vi "IntPRFCount.vi"(0 "prf (kHz)":dbl=1.0 format="%.3f", 2 "prf (f)/motor (t)":bool, 9 "Divide prf by":i32=2, 13 "therapy divide by (T)":bool) -> (6 "new prf":dbl format="%.2f", 15 "Divide prf out":i32=1)   [LabVIEW 2022 SP3]
uses:
  Pulsers/PulserGlobals.vi
  Motion Controllers/-MotionRoutines/MotionGlobals.vi
  <vilib>/DAQmx/create/channels.llb/DAQmx Create Channel (CO-Pulse Generation-Ticks).vi
  <vilib>/DAQmx/create/channels.llb/DAQmx Create Channel (CO-Pulse Generation-Frequency).vi
panel:
  # "Indicates if counter 0 is is giving a 1-1 output pulse\n for each motor inpute or if it is generating a continous prf."
  # "Determines whether counter 1 is used to fire \ntherapy at some divided multiple of counter 0."
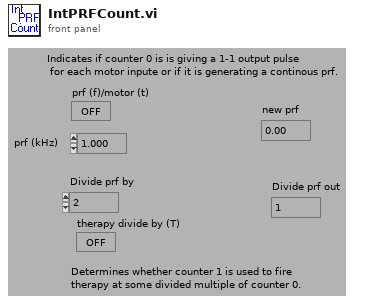
[diagram p1: front panel]
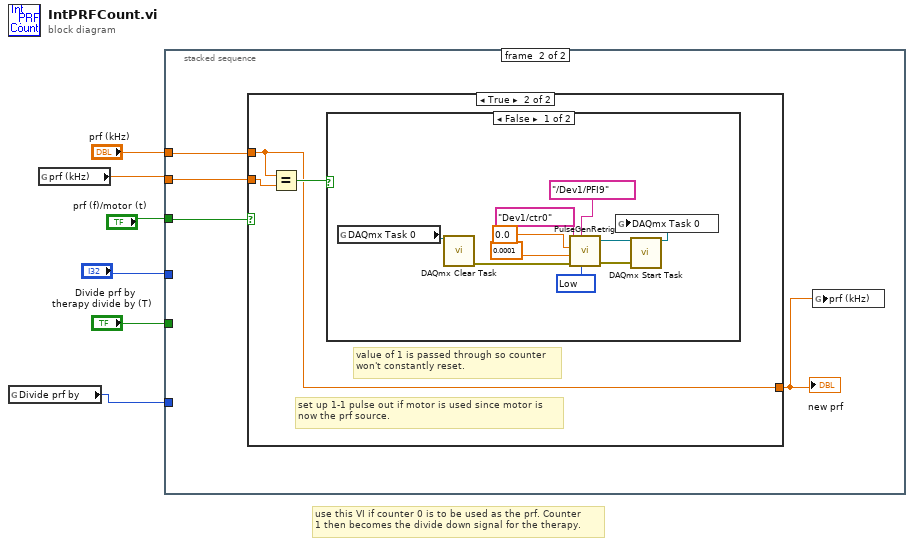
[diagram p0: block diagram]
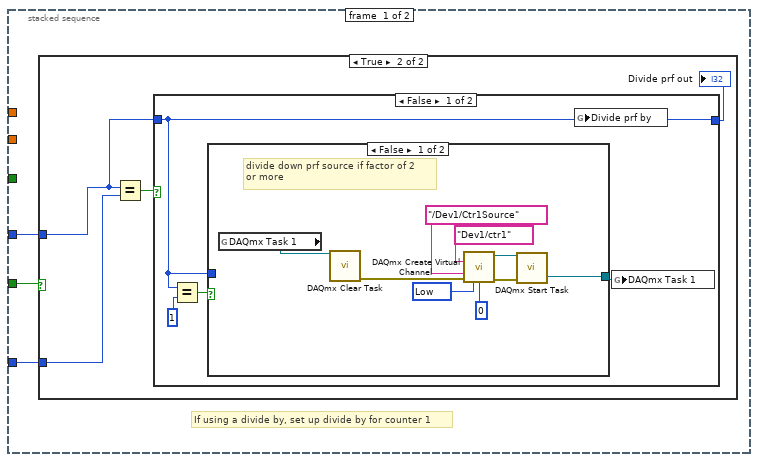
[diagram p2: hidden frame]
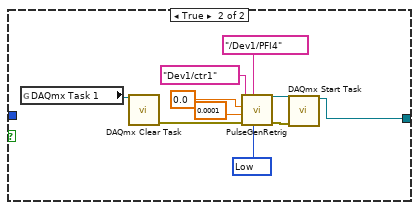
[diagram p4: hidden frame]
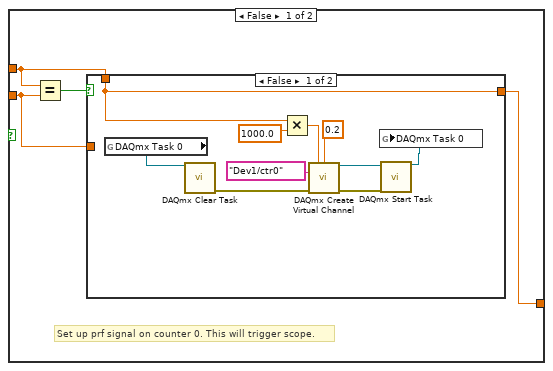
[diagram p6: hidden frame]
diagram:
  # "use this VI if counter 0 is to be used as the prf. Counter\n1 then becomes the divide down signal for the therapy."
  n1 = global read "PulserGlobals.vi" "Divide prf by"() -> (w2:i32)
  n2 = global read "PulserGlobals.vi" "prf (kHz)"() -> (w1:dbl)
  n3 = stacked-sequence {
    tunnel: "prf (kHz)" -> [_ w41]
    tunnel: w1 -> [_ w40]
    tunnel: "therapy divide by (T)" -> [w9 _]
    tunnel: w2 -> [w8 _]
    tunnel: "prf (f)/motor (t)" -> [_ w39]
    tunnel: "Divide prf by" -> [w7 _]
    frame #0 {
      # "If using a divide by, set up divide by for counter 1"
      n4 = case shown="True" w9 {
        tunnel: w8 -> [_ w10]
        tunnel: w7 -> [_ w12]
        frame False {
        }
        frame True {
          n5 = Equal?(x=w12, y=w10) -> (x = y?=w13:bool)
          n6 = case shown="False" w13 {
            tunnel: [w14 w37] -> w11
            tunnel: w12 -> [w14 w37]
            frame False {
              n7 = Equal?(x=w14, y=1) -> (x = y?=w16:bool)
              n8 = case shown="False" w16 {
                tunnel: w14 -> [_ _]
                tunnel: [w26 w36] -> w15
                frame False {
                  w18 = 10214 items=["High"=10192, "Low"=10214] ("idle state")
                  # "divide down prf source if factor of 2 \nor more"
                  n9 = global read "MotionGlobals.vi" "DAQmx Task 1"() -> (w24:refnum<k21>)
                  n10 = call <vilib>:"DAQmx Clear Task.vi"("task in"=w24) -> ("error out"=w25:errorcluster)  [unwired: 1 in, 13 out]
                  n11 = call-poly <vilib>:"DAQmx Create Virtual Channel.vi"("counter"=tag "Dev1/ctr1", "source of ticks"=tag "/Dev1/Ctr1Source", "error in"=w25, "idle state"=w18, "initial delay"=0) -> ("task out"=w20:refnum<k21>, "error out"=w19:errorcluster)  [unwired: 4 in, 5 out]
                  n12 = call <vilib>:"DAQmx Start Task.vi"("task/channels in"=w20, "error in"=w19) -> ("task out"=w26:refnum<k21>)  [unwired: 13 out]
                }
                frame True {
                  w31 = 10214 items=["High"=10192, "Low"=10214] ("idle state")
                  n13 = global read "MotionGlobals.vi" "DAQmx Task 1"() -> (w34:refnum<k21>)
                  n14 = call <vilib>:"DAQmx Clear Task.vi"("task in"=w34) -> ("error out"=w35:errorcluster)  [unwired: 1 in, 13 out]
                  n15 = call "PulseGenRetrig.vi"("idle state"=w31, "source"=tag "/Dev1/PFI4", "error in"=w35, "high time"=0.0001, "pulse delay (s or cycles)"=0.0, "counter"=tag "Dev1/ctr1") -> ("error out"=w28:errorcluster, "task out"=w29:refnum<k21>)
                  n16 = call <vilib>:"DAQmx Start Task.vi"("task/channels in"=w29, "error in"=w28) -> ("task out"=w36:refnum<k21>)  [unwired: 13 out]
                }
              }
              n17 = global write "PulserGlobals.vi" "Divide prf by"(w14) -> ()
              n18 = global write "MotionGlobals.vi" "DAQmx Task 1"(w15) -> ()
            }
            frame True {
            }
          }
          "Divide prf out" <- w11
        }
      }
    }
    frame #1 {
      n19 = case shown="True" w39 {
        tunnel: w41 -> [w44 w58]
        tunnel: w40 -> [w43 w57]
        tunnel: [w42 w58] -> w38
        frame False {
          # "Set up prf signal on counter 0. This will trigger scope."
          n20 = Equal?(x=w44, y=w43) -> (x = y?=w45:bool)
          n21 = case shown="False" w45 {
            tunnel: w44 -> [w55 _]
            tunnel: [w55 w56] -> w42
            tunnel: w43 -> [_ w56]
            frame False {
              n22 = global read "MotionGlobals.vi" "DAQmx Task 0"() -> (w53:refnum<k21>)
              n23 = call <vilib>:"DAQmx Clear Task.vi"("task in"=w53) -> ("error out"=w54:errorcluster)  [unwired: 1 in, 13 out]
              n24 = Multiply(x=w55, y=1000.0) -> (x*y=w48:dbl)
              n25 = call-poly <vilib>:"DAQmx Create Virtual Channel.vi"("frequency"=w48, "duty cycle"=0.2, "counter"=tag "Dev1/ctr0", "error in"=w54) -> ("task out"=w51:refnum<k21>, "error out"=w50:errorcluster)  [unwired: 5 in, 5 out]
              n26 = call <vilib>:"DAQmx Start Task.vi"("task/channels in"=w51, "error in"=w50) -> ("task out"=w46:refnum<k21>)  [unwired: 13 out]
              n27 = global write "MotionGlobals.vi" "DAQmx Task 0"(w46) -> ()
            }
            frame True {
            }
          }
        }
        frame True {
          # "value of 1 is passed through so counter\nwon't constantly reset."
          # "set up 1-1 pulse out if motor is used since motor is\nnow the prf source."
          n28 = Equal?(x=w58, y=w57) -> (x = y?=w59:bool)
          n29 = case shown="False" w59 {
            frame False {
              w65 = 10214 items=["High"=10192, "Low"=10214] ("idle state")
              n30 = global read "MotionGlobals.vi" "DAQmx Task 0"() -> (w68:refnum<k21>)
              n31 = call <vilib>:"DAQmx Clear Task.vi"("task in"=w68) -> ("error out"=w69:errorcluster)  [unwired: 1 in, 13 out]
              n32 = call "PulseGenRetrig.vi"("idle state"=w65, "source"=tag "/Dev1/PFI9", "error in"=w69, "high time"=0.0001, "pulse delay (s or cycles)"=0.0, "counter"=tag "Dev1/ctr0") -> ("error out"=w63:errorcluster, "task out"=w64:refnum<k21>)
              n33 = call <vilib>:"DAQmx Start Task.vi"("task/channels in"=w64, "error in"=w63) -> ("task out"=w61:refnum<k21>)  [unwired: 13 out]
              n34 = global write "MotionGlobals.vi" "DAQmx Task 0"(w61) -> ()
            }
            frame True {
            }
          }
        }
      }
      "new prf" <- w38
      n35 = global write "PulserGlobals.vi" "prf (kHz)"(w38) -> ()
    }
  }
